vi "Dotted Name to Index.vi"(10 "Item Graph":T1[](array[typedef]), 11 "Dotted Name":string) -> (3 "Index":i32)   [LabVIEW 2016, in "Better Search.lvlib"]
uses:
  Better Search.lvlib
  Data Types/Type Reflection Item.ctl
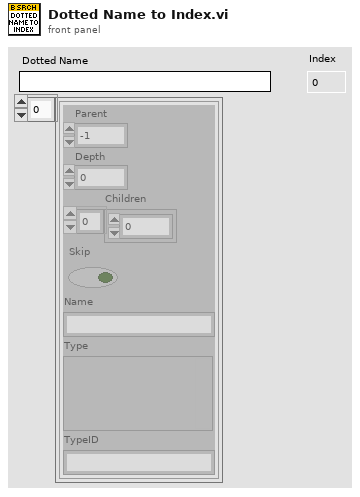
[diagram p1: front panel]
types:
  T1 = typedef "Better Search.lvlib/Type Reflection Item.ctl" = cluster{"Parent":i32, "Depth":i32, "Children":i32[], "Skip":bool, "Name":string, "Type":variant, "TypeID":string}
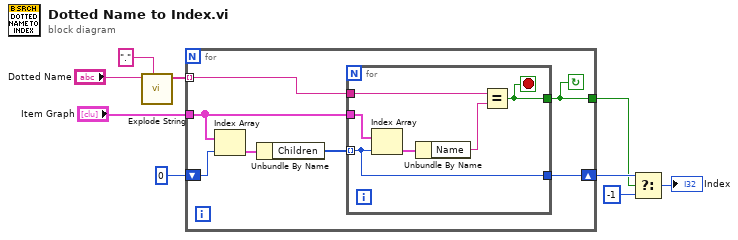
[diagram p0: block diagram]
diagram:
  n1 = call "Explode String.vi"("Delimiter (Comma)"="." ("delimiter"), "Delimited String"="Dotted Name") -> ("String Array"=w2:string[])  [unwired: 9 in]
  n2 = for {
    tunnel: w2 -> [w12] mode=indexing
    tunnel: "Item Graph" -> [w13]
    shift-right: [w11] -> w7
    shift-left: 0 -> [w16]
    tunnel: [w10] -> w4
    stop <- w10 continue-if-true
    n3 = Index Array(array=w13, index=w16) -> (element=w15:T1)
    n4 = Unbundle By Name(w15) -> ("Children"=w14:i32[])
    n5 = for {
      tunnel: w14 -> [w18] mode=indexing
      tunnel: w13 -> [w22]
      tunnel: w12 -> [w19]
      tunnel: [w18] -> w11
      tunnel: [w17] -> w10
      stop <- w17 stop-if-true
      n6 = Index Array(array=w22, index=w18) -> (element=w21:T1)
      n7 = Unbundle By Name(w21) -> ("Name"=w20:string)
      n8 = Equal?(x=w19, y=w20) -> (x = y?=w17:bool)
    }
  }
  n9 = Select(t=w7, s=w4, f=-1) -> (s? t:f=→"Index":i32)
